vi "Format Item Name.vi"(8 "error in (no error)":errorcluster, 9 "Flat View?":bool, 10 "Abbreviate Names?":bool, 11 "Item in":refnum<class "Item.lvclass">) -> (0 "error out":errorcluster, 3 "Item out":refnum<class "Item.lvclass">)   [LabVIEW 2020, in "VI Properties Editor.lvlib" / "Item.lvclass"]
doc: "Formats the item names to be displayed, based on <B>Abbreviate Names?</B>, <B>Flat View</B>, and if modifications have been made."
uses:
  Item.lvclass
  <vilib>/AdvancedString/Delimited String to 1D String Array (string).vi
  VI Properties Editor.lvlib
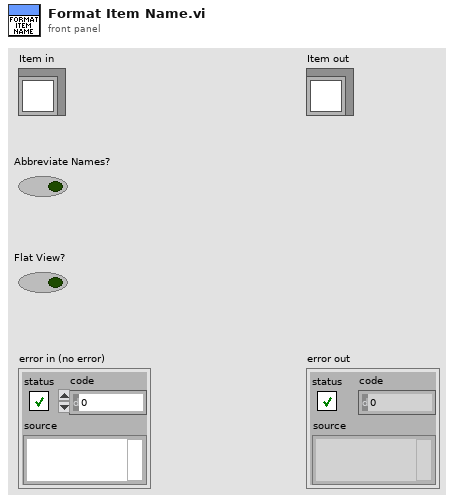
[diagram p1: front panel]
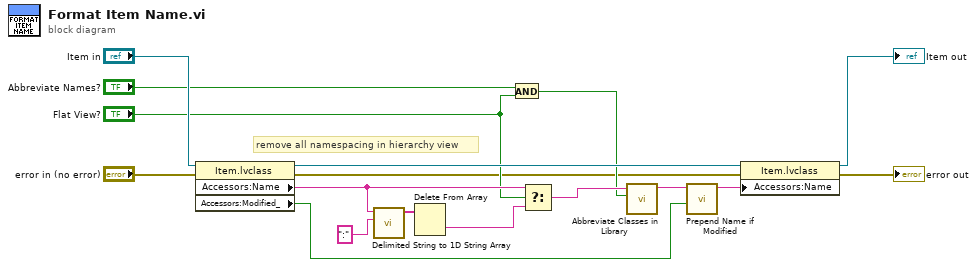
[diagram p0: block diagram]
diagram:
  # "remove all namespacing in hierarchy view"
  n1 = property class="Item.lvclass"(reference="Item in", error in="error in (no error)") -> (reference out=w17:refnum<class "Item.lvclass">, error out=w2:errorcluster, "Accessors:Name"=w14:string, "Accessors:Modified_"=w9:bool)
  n2 = call-poly <vilib>:"Delimited String to 1D String Array.vi"("delimiter"=":", "delimited string"=w14) -> ("string array"=w16:string[])  [unwired: 9 in]
  n3 = Delete From Array(array=w16) -> (deleted portion=w13:string)  [unwired: 2 in, 1 out]
  n4 = And(x="Abbreviate Names?", y="Flat View?") -> (x .and. y?=w5:bool)
  n5 = Select(t=w14, s="Flat View?", f=w13) -> (s? t:f=w12:string)
  n6 = call "Abbreviate Classes in Library.vi"("Abbreviate Name?"=w5, "Name"=w12) -> ("Name out"=w11:string)  [unwired: 9 in]
  n7 = call "Prepend Name if Modified.vi"("Modified?"=w9, "VI Name"=w11) -> ("VI Name out"=w10:string)  [unwired: 9 in]
  n8 = property class="Item.lvclass"(reference=w17, error in=w2, "Accessors:Name"=w10) -> (reference out=→"Item out":refnum<class "Item.lvclass">, error out=→"error out":errorcluster)
